vi "Get Plot at Mouse Click in Plot Area [AAC].vi"(8 "error in (no error)":errorcluster, 10 "Mouse Click Coordinates (defaut: last plot)":T2={"Horizontal"=2147483647, "Vertical"=0}, 11 "XYGraph Ref":T1) -> (0 "error out":errorcluster, 1 "Plot Index":i32, 3 "XYGraph Ref":T1)   [LabVIEW 2021, in "Graphs.lvlib"]
doc: "If the Mouse Coordinates X value = 2147483647 (max I32 value), this means that the last plot is sought for is thus the plot returned.\nIf there is no plot in the Graph, -1 is returned"
uses:
  Graphs.lvlib
  XY Graph/XY Graph Refnum.ctl
  <vilib>/Utility/miscctls.llb/LVPoint32TypeDef.ctl
  XY Graph/XY Graph Add-Ons.lvlib
panel:
  in  "Array of Array Cluster":cluster{"Array":dbl[], "Array":dbl[]}[](array[cluster])
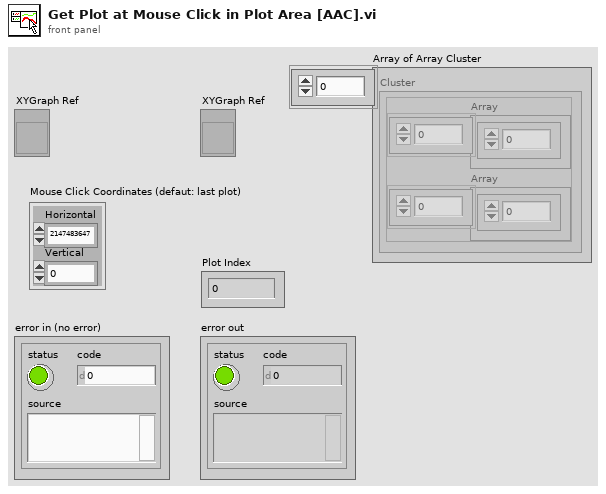
[diagram p1: front panel]
types:
  T1 = typedef "XY Graph Add-Ons.lvlib/XY Graph Refnum.ctl" = refnum<vi>
  T2 = typedef "LVPoint32TypeDef.ctl" = cluster{"Horizontal":i32, "Vertical":i32}
  T3 = typedef "LVRectTypeDef.ctl" = cluster{"Left":i16, "Top":i16, "Right":i16, "Bottom":i16}
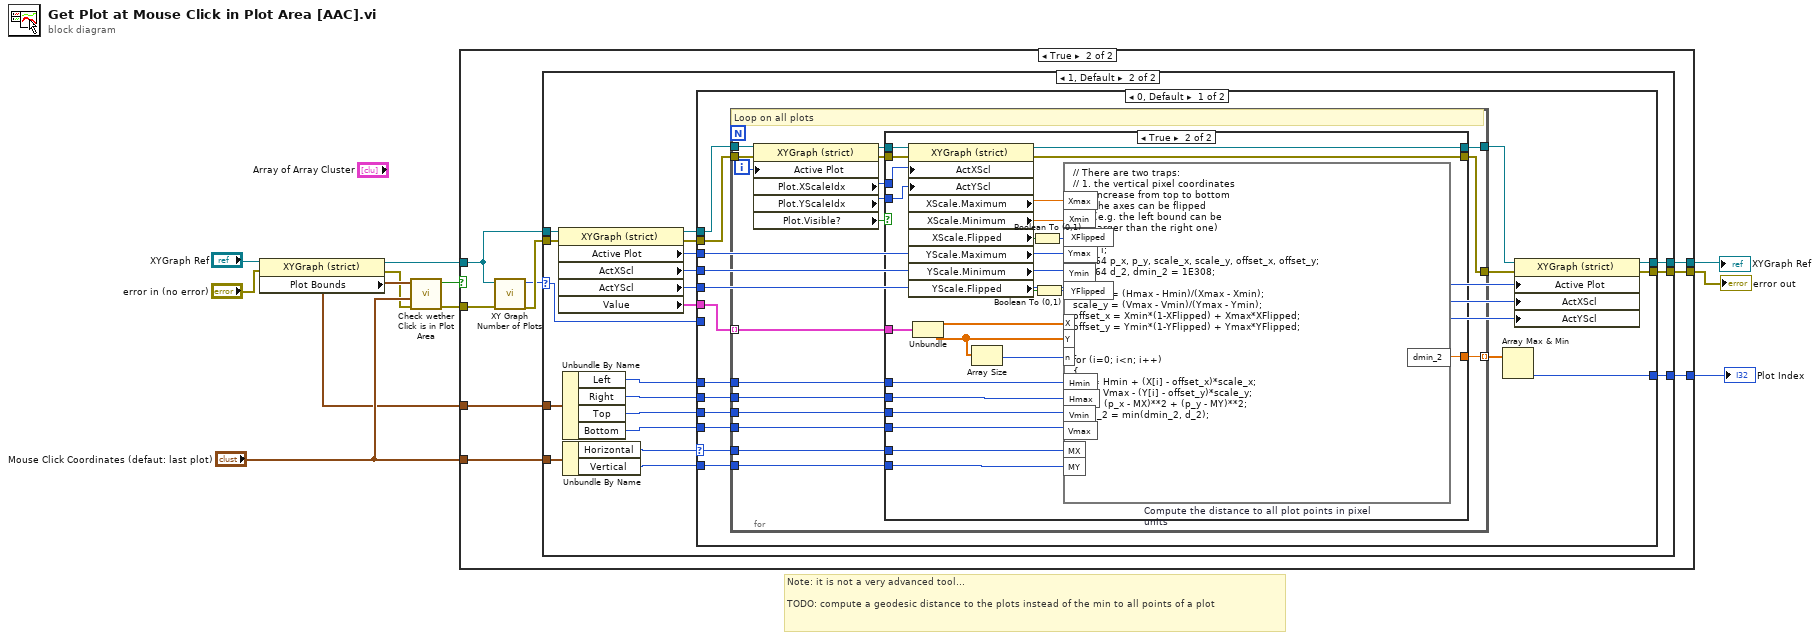
[diagram p0: block diagram]
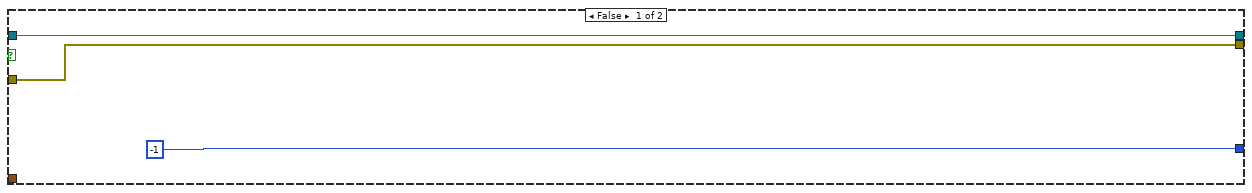
[diagram p2: hidden frame]
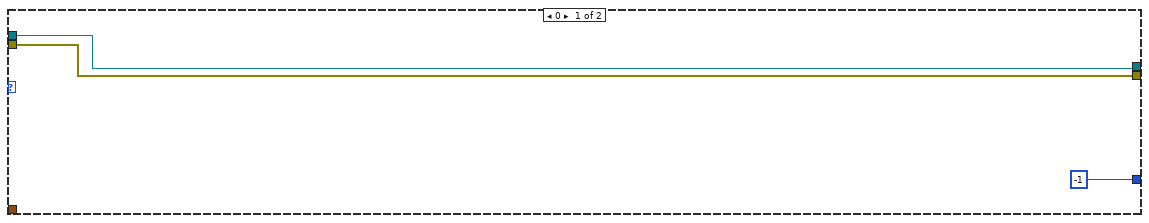
[diagram p3: hidden frame]
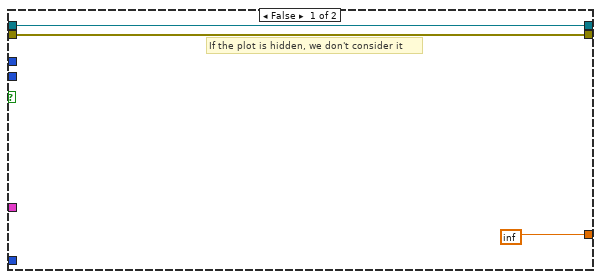
[diagram p4: hidden frame]
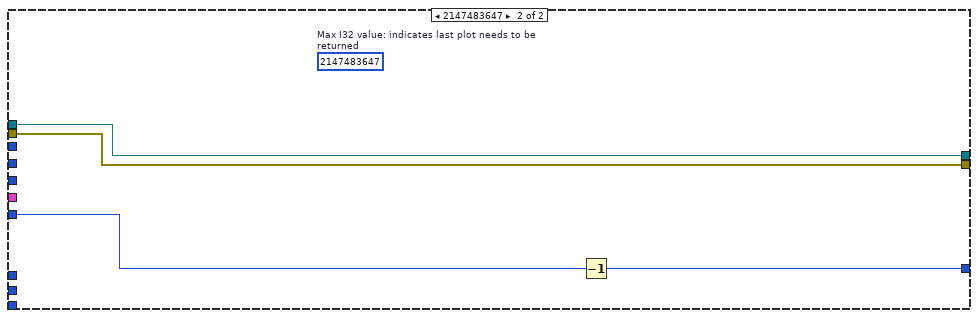
[diagram p5: hidden frame]
diagram:
  # "Note: it is not a very advanced tool...\n\nTODO: compute a geodesic distance to the plots instead of the min to all points of a plot"
  n1 = property class="XYGraph (strict)"(reference="XYGraph Ref", error in="error in (no error)") -> (reference out=w8:T1, error out=w2:errorcluster, "Plot Bounds"=w3:T3)
  n2 = call "Check wether Click is in Plot Area.vi"("Error In"=w2, "Mouse Click Coordinates"="Mouse Click Coordinates (defaut: last plot)", "Plot Bounds"=w3) -> ("Error Out"=w1:errorcluster, "Is in Plot Area?"=w9:bool)  [unwired: 7 in]
  n3 = case shown="True" w9 {
    tunnel: w8 -> [w14 w18]
    tunnel: [w14 w23] -> w7
    tunnel: [w12 w22] -> w6
    tunnel: [-1 ("Plot Index") w19] -> w5
    tunnel: "Mouse Click Coordinates (defaut: last plot)" -> [_ w21]
    tunnel: w3 -> [_ w20]
    tunnel: w1 -> [w12 w15]
    frame False {
    }
    frame True {
      n4 = call "XY Graph Number of Plots.vi"("Error In"=w15, "XYGraph in"=w18) -> ("Error Out"=w17:errorcluster, "# Plots"=w16:i32)  [unwired: 8 in]
      n5 = case shown="1, Default" w16 {
        selector: w16 -> [_ w27]
        tunnel: [w25 w46] -> w23
        tunnel: [w24 w45] -> w22
        tunnel: w21 -> [_ w44]
        tunnel: w20 -> [_ w43]
        tunnel: [-1 w42] -> w19
        tunnel: w18 -> [w25 w30]
        tunnel: w17 -> [w24 w29]
        frame 0 {
        }
        frame 1, Default {
          n6 = property class="XYGraph (strict)"(reference=w30, error in=w29) -> (reference out=w41:T1, error out=w28:errorcluster, "Active Plot"=w40:u32, "ActXScl"=w39:i32, "ActYScl"=w38:i32, "Value"=w31:cluster{"X Array":dbl[], "Y Array":dbl[]}[])
          n7 = Unbundle By Name(w43) -> ("Left"=w37:i16, "Right"=w36:i16, "Top"=w35:i16, "Bottom"=w34:i16)
          n8 = Unbundle By Name(w44) -> ("Horizontal"=w33:i32, "Vertical"=w32:i32)
          n9 = case shown="0, Default" w33 {
            selector: w33 -> [w53 _]
            tunnel: [w64 w112] -> w46
            tunnel: [w63 w111] -> w45
            tunnel: [w62 w113] -> w42
            tunnel: w41 -> [w61 w112]
            tunnel: w40 -> [w60 _]
            tunnel: w39 -> [w59 _]
            tunnel: w38 -> [w58 _]
            tunnel: w37 -> [w57 _]
            tunnel: w36 -> [w56 _]
            tunnel: w35 -> [w55 _]
            tunnel: w34 -> [w54 _]
            tunnel: w32 -> [w52 _]
            tunnel: w31 -> [w51 _]
            tunnel: w28 -> [w48 w111]
            tunnel: w27 -> [_ w114]
            frame 0, Default {
              n10 = for {
                tunnel: w51 -> [w82] mode=indexing
                tunnel: w61 -> [w69]
                tunnel: [w77] -> w50
                tunnel: w57 -> [w76]
                tunnel: w56 -> [w75]
                tunnel: w55 -> [w74]
                tunnel: w54 -> [w73]
                tunnel: w53 -> [w72]
                tunnel: w52 -> [w71]
                tunnel: [w70] -> w49 mode=indexing
                tunnel: w48 -> [w67]
                tunnel: [w65] -> w47
                i -> [w81]
                # "Loop on all plots"
                n11 = property class="XYGraph (strict)"(reference=w69, error in=w67, "Active Plot"=w81) -> (reference out=w80:T1, error out=w66:errorcluster, "Plot.XScaleIdx"=w79:u32, "Plot.YScaleIdx"=w78:u32, "Plot.Visible?"=w68:bool)
                n12 = case shown="True" w68 {
                  tunnel: w82 -> [_ w110]
                  tunnel: w80 -> [w85 w109]
                  tunnel: w79 -> [_ w108]
                  tunnel: w78 -> [_ w107]
                  tunnel: [w85 w106] -> w77
                  tunnel: w76 -> [_ w101]
                  tunnel: w75 -> [_ w100]
                  tunnel: w74 -> [_ w99]
                  tunnel: w73 -> [_ w98]
                  tunnel: w72 -> [_ w97]
                  tunnel: w71 -> [_ w96]
                  tunnel: [inf w94] -> w70
                  tunnel: w66 -> [w83 w87]
                  tunnel: [w83 w86] -> w65
                  frame False {
                    # "If the plot is hidden, we don't consider it"
                  }
                  frame True {
                    n13 = property class="XYGraph (strict)"(reference=w109, error in=w87, "ActXScl"=w108, "ActYScl"=w107) -> (reference out=w106:T1, error out=w86:errorcluster, "XScale.Maximum"=w105:dbl, "XScale.Minimum"=w104:dbl, "XScale.Flipped"=w93:bool, "YScale.Maximum"=w103:dbl, "YScale.Minimum"=w102:dbl, "YScale.Flipped"=w91:bool)
                    n14 = Unbundle(w110) -> ("X Array"=w95:dbl[], "Y Array"=w89:dbl[])
                    n15 = Array Size(array=w89) -> (size(s)=w88:i32)
                    n16 = Boolean To (0,1)(Boolean=w93) -> (0, 1=w92:i16)
                    n17 = Boolean To (0,1)(Boolean=w91) -> (0, 1=w90:i16)
                    n18 = formula code="// There are two traps:\n// 1. the vertical pixel coordinates\n//     increase from top to bottom\n// 2. the axes can be flipped\n//     (e.g. the left bound can be\n//     larger than the right one)\n\nint32 i;\nfloat64 p_x, p_y, scale_x, scale_y, offset_x, offset_y;\nfloat64 d_2, dmin_2 = 1E308;\n\nscale_x = (Hmax - Hmin)/(Xmax - Xmin);\nscale_y = (Vmax - Vmin)/(Ymax - Ymin);\noffset_x = Xmin*(1-XFlipped) + Xmax*XFlipped;\noffset_y = Ymin*(1-YFlipped) + Ymax*YFlipped;\n\n\nfor (i=0; i<n; i++)\n{\np_x = Hmin + (X[i] - offset_x)*scale_x;\np_y = Vmax - (Y[i] - offset_y)*scale_y;\nd_2 = (p_x - MX)**2 + (p_y - MY)**2;\ndmin_2 = min(dmin_2, d_2);\n}" "Compute the distance to all plot points in pixel units"("Xmax"=w105, "Xmin"=w104, "Ymax"=w103, "Ymin"=w102, "Hmin"=w101, "Hmax"=w100, "Vmin"=w99, "Vmax"=w98, "MX"=w97, "MY"=w96, "X"=w95, "Y"=w89, "XFlipped"=w92, "YFlipped"=w90, "n"=w88) -> ("dmin_2"=w94:dbl)
                  }
                }
              }
              n19 = Array Max & Min(array=w49) -> (min index (indices)=w62:i32)  [unwired: 3 out]
              n20 = property class="XYGraph (strict)"(reference=w50, error in=w47, "Active Plot"=w60, "ActXScl"=w59, "ActYScl"=w58) -> (reference out=w64:T1, error out=w63:errorcluster)
            }
            frame 2147483647 {
              (unwired) 2147483647  # Max I32 value: indicates last plot needs to be returned
              n21 = Decrement(x=w114) -> (x-1=w113:i32)
            }
          }
        }
      }
    }
  }
  "Plot Index" <- w5
  "XYGraph Ref" <- w7
  "error out" <- w6
